vi "Update_bottle_selection.vi"(5 "Position":T5, 7 "Bounds":T4, 8 "Coords":T3, 9 "Odour bottles in":T2(array[cluster])) -> (0 "selected bottle":T1, 3 "Odour bottles out":T2(array[cluster]))   [LabVIEW 2016]
uses:
  <vilib>/Utility/miscctls.llb/LVPositionTypeDef.ctl
  <vilib>/Utility/miscctls.llb/LVBoundsTypeDef.ctl
  <vilib>/Utility/miscctls.llb/LVPoint32TypeDef.ctl
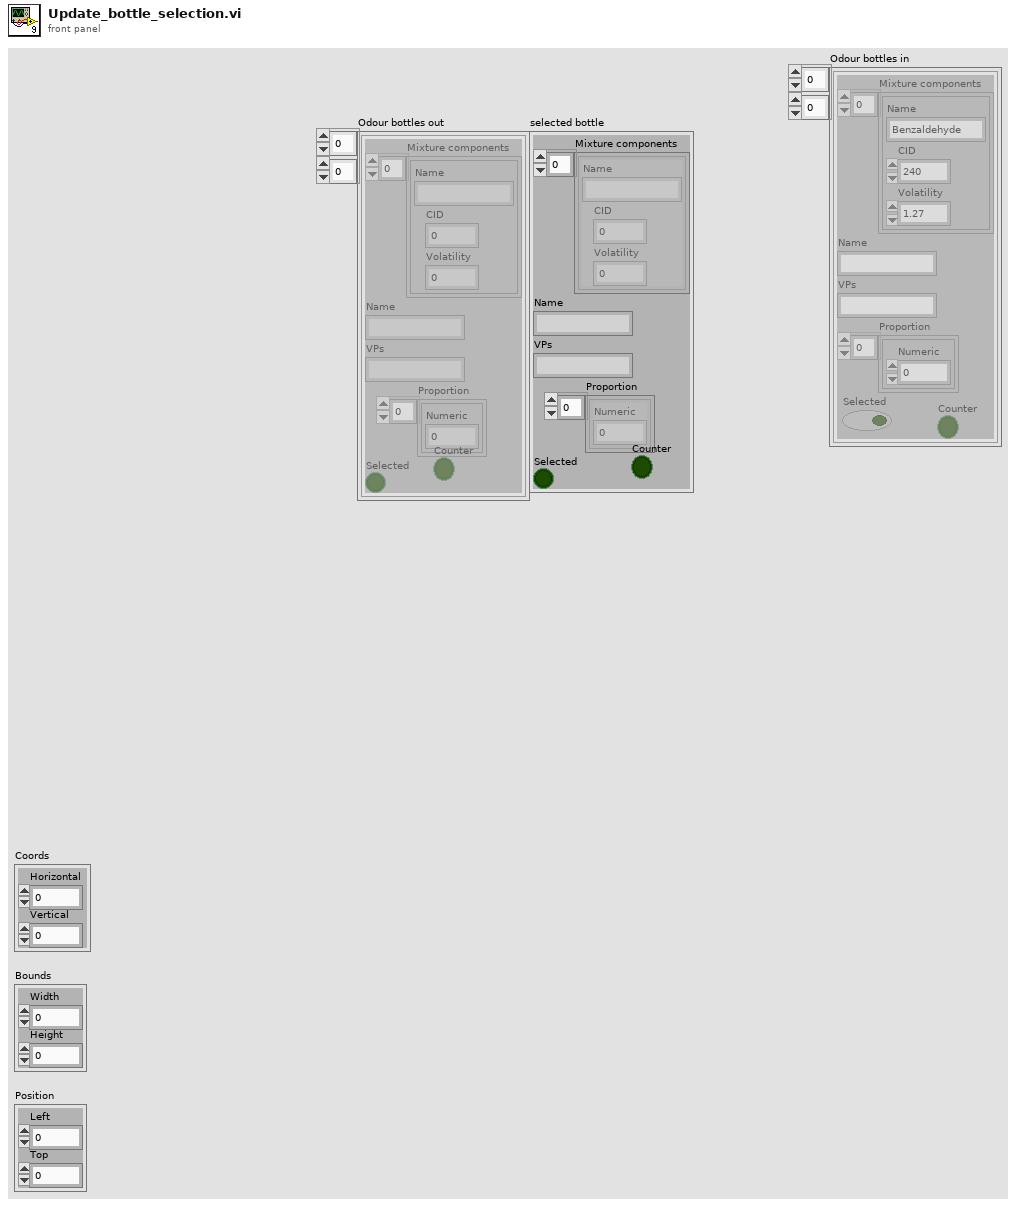
[diagram p1: front panel]
types:
  T1 = cluster{"Mixture components":cluster{"Name":string, "CID":i32, "Volatility":dbl}[], "Name":string, "VPs":string, "Proportion":cluster{"Numeric":dbl}[], "Selected":bool, "Counter":bool}
  T2 = cluster{"Mixture components":cluster{"Name":string, "CID":i32, "Volatility":dbl}[], "Name":string, "VPs":string, "Proportion":cluster{"Numeric":dbl}[], "Selected":bool, "Counter":bool}[][]
  T3 = typedef "LVPoint32TypeDef.ctl" = cluster{"Horizontal":i32, "Vertical":i32}
  T4 = typedef "LVBoundsTypeDef.ctl" = cluster{"Width":u32, "Height":u32}
  T5 = typedef "LVPositionTypeDef.ctl" = cluster{"Left":i32, "Top":i32}
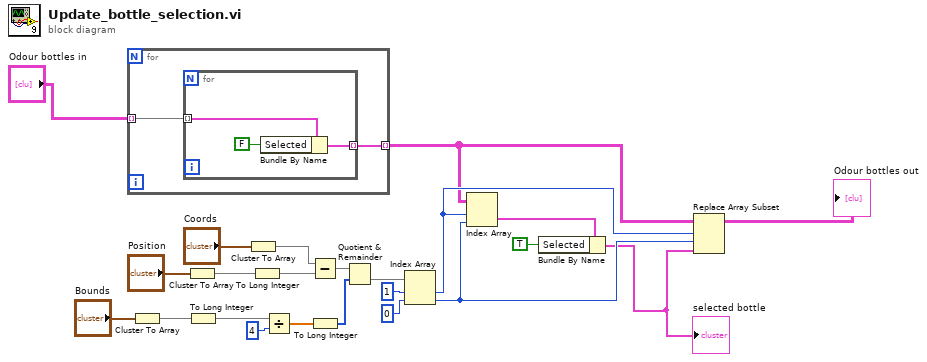
[diagram p0: block diagram]
diagram:
  n1 = for {
    tunnel: "Odour bottles in" -> [w25] mode=indexing
    tunnel: [w24] -> w17 mode=indexing
    n2 = for {
      tunnel: w25 -> [w28] mode=indexing
      tunnel: [w27] -> w24 mode=indexing
      n3 = Bundle By Name(cluster=w28, "Selected"=FALSE) -> (w27:T1)
    }
  }
  n4 = Cluster To Array(cluster="Bounds") -> (array=w4:u32[])
  n5 = Cluster To Array(cluster="Position") -> (array=w3:i32[])
  n6 = To Long Integer(number=w4) -> (32bit integer=w5:i32[])
  n7 = Cluster To Array(cluster="Coords") -> (array=w6:i32[])
  n8 = To Long Integer(number=w3) -> (32bit integer=w7:i32[])
  n9 = Divide(x=w5, y=4) -> (x/y=w9:dbl[])
  n10 = Subtract(x=w6, y=w7) -> (x-y=w8:i32[])
  n11 = To Long Integer(number=w9) -> (32bit integer=w10:i32[])
  n12 = Quotient & Remainder(x=w8, y=w10) -> (floor(x/y)=w21:i32[])  [unwired: 1 out]
  n13 = Index Array(array=w21, index #1=1 ("index"), index #2=0 ("index")) -> (element #1=w23:i32, element #2=w22:i32)
  n14 = Index Array(array=w17, index (row)=w23, index (col)=w22) -> (element=w18:T1)
  n15 = Bundle By Name(cluster=w18, "Selected"=TRUE) -> (w20:T1)
  "selected bottle" <- w20
  n16 = Replace Array Subset(array=w17, new element=w20, index (row)=w23, index (col)=w22) -> (→"Odour bottles out":T2)
